vi "CMI ADS127L21 - Config Input.vi"(5 "Range [Vpk]":dbl, 7 "Impedance":T2, 8 "error in (no error)":errorcluster, 9 "Mode":T1, 10 "channel id (1: first)":i32, 11 "session in":T3 {"channels"."Channel" min=1 max=8 step=1; "channels"."Range [Vpk]" items=["±1.65V", "±2V"]}) -> (0 "error out":errorcluster, 3 "session out":T3 {"channels"."Channel" min=1 max=8 step=1; "channels"."Range [Vpk]" items=["±1.65V", "±2V"]})   [LabVIEW 2020]
doc: "Config input channel."
uses:
  CMI ADS127L21 - Session.ctl
  CMI ADS127L21 - Record Channel.ctl
  CMI ADS127L21 - Input Range.ctl
  CMI ADS127L21 - Input Mode.ctl
  CMI ADS127L21 - Input Impedance.ctl
  CMI ADS127L21 - EXTOUT Mode.ctl
  CMI ADS127L21 - EXTOUT Polarity.ctl
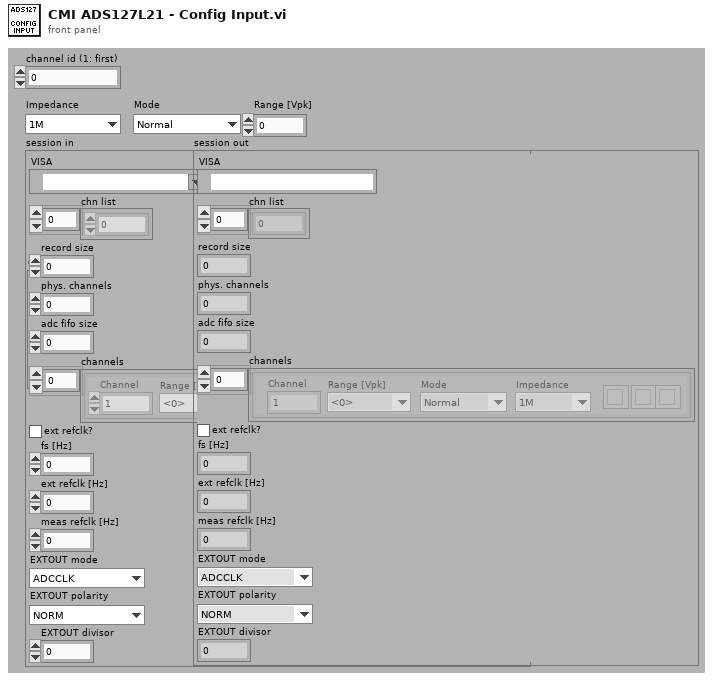
[diagram p1: front panel]
types:
  T1 = typedef "CMI ADS127L21 - Input Mode.ctl" = enum16{"Normal", "Inverted", "GND"}
  T2 = typedef "CMI ADS127L21 - Input Impedance.ctl" = enum16{"1M", "1k5"}
  T3 = typedef "CMI ADS127L21 - Session.ctl" = cluster{"VISA":refnum<visa-resource-name>, "chn list":i32[], "record size":i32, "phys. channels":i32, "adc fifo size":i32, "channels":T4[], "ext refclk?":bool, "fs [Hz]":dbl, "ext refclk [Hz]":dbl, "meas refclk [Hz]":dbl, "EXTOUT mode":T6, "EXTOUT polarity":T7, "EXTOUT divisor":i32}
  T4 = typedef "CMI ADS127L21 - Record Channel.ctl" = cluster{"Range [Vpk]":T5, "Channel":i32, "Mode":T1, "Impedance":T2, "btn clr":bool, "btn up":bool, "btn down":bool}
  T5 = typedef "CMI ADS127L21 - Input Range.ctl" = dbl
  T6 = typedef "CMI ADS127L21 - EXTOUT Mode.ctl" = enum16{"ADCCLK", "REFCLK", "SMPLCLK", "FIRST"}
  T7 = typedef "CMI ADS127L21 - EXTOUT Polarity.ctl" = enum16{"NORM", "INV"}
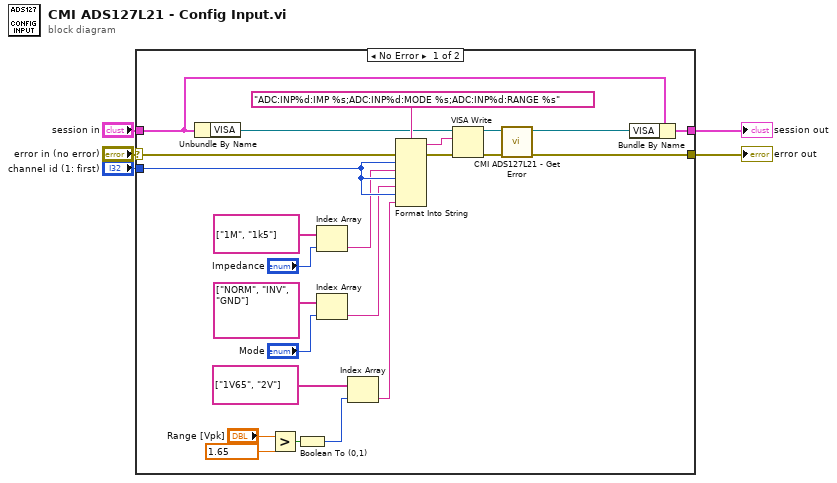
[diagram p0: block diagram]
diagram:
  n1 = case shown="No Error" "error in (no error)" {
    selector: "error in (no error)" -> [w13 w31]
    tunnel: "channel id (1: first)" -> [w26 _]
    tunnel: "session in" -> [w10 w30]
    tunnel: [w11 w30] -> w3
    tunnel: [w14 w31] -> w2
    frame No Error {
      w7 = T5 1.65 items=["±1.65V"=1.65, "±2V"=2.0] ("y")
      n2 = Unbundle By Name(w10) -> ("VISA"=w12:refnum<visa-resource-name>)
      n3 = Greater?(x="Range [Vpk]", y=w7) -> (0:w8:bool)
      n4 = Boolean To (0,1)(Boolean=w8) -> (0, 1=w6:i16)
      n5 = Index Array(array=string[] ["1M", "1k5"], index="Impedance") -> (element=w25:string)
      n6 = Index Array(array=string[] ["NORM", "INV", "GND"], index="Mode") -> (element=w22:string)
      n7 = Index Array(array=string[] ["1V65", "2V"], index=w6) -> (element=w20:string)
      n8 = Format Into String(format string="ADC:INP%d:IMP %s;ADC:INP%d:MODE %s;ADC:INP%d:RANGE %s", error in=w13, w26, w25, w26, w22, w26, w20) -> (resulting string=w16:string, error out=w19:errorcluster)  [unwired: 1 in]
      n9 = VISA Write(VISA resource name=w12, write buffer=w16, error in (no error)=w19) -> (VISA resource name out=w17:refnum<visa-resource-name>, error out=w18:errorcluster)  [unwired: 1 out]
      n10 = call "CMI ADS127L21 - Get Error.vi"("error in (no error)"=w18, "VISA in"=w17) -> ("error out"=w14:errorcluster, "VISA out"=w15:refnum<visa-resource-name>)  [unwired: 8 in]
      n11 = Bundle By Name(cluster=w10, "VISA"=w15) -> (w11:T3)
    }
    frame Error {
    }
  }
  "error out" <- w2
  "session out" <- w3
